vi "Update_Data_Packet_From_Processed_Bytes_Receiver.vi"(0 "Processed Bytes":u8[](array[numeric]), 1 "Receive count":u32, 2 "Receive interval (ms)":u32, 5 "Last Receive Time (ms)":u64, 11 "error in (no error)":errorcluster) -> (4 "Updated data packet":T1={"Packet"={"Raw Bytes"=[], "Checksum"=FALSE, "Direction"=enum."Transmit", "Processed Bytes"=[], "Node ID"=0, "Packet type"=enum."Connection Management", "Frame Data"=0, "Priority"=enum."LOW", "Frame ID"=0}, "Parameters"=[], "Last Received Time (ms)"=0, "Receive count"=0, "Transmit count"=0, "Transmit interval (ms)"=0, "Last Transmitted Time (ms)"=0, "Receive interval (ms)"=0, "Transmit_Mode"=enum."Disabled", "Transmit Enable"=FALSE, "Cyclic Transmit interval (ms)"=0}, 6 "Data Packets Out":T1[](array[typedef]), 15 "error out":errorcluster)   [LabVIEW 2017]
uses:
  Controls/Data Packets/Data_Packet.ctl
  Controls/Packet/Packet.ctl
  Controls/Packet/Packet_Direction.ctl
  Controls/Packet/Packet_Type.ctl
  Controls/Packet/Packet_Priority.ctl
  Controls/Data Packets/Parameter.ctl
  Controls/Data Packets/Parameter_Data_Type.ctl
  Controls/Data Packets/Data_Packet_Transmit_Mode.ctl
  Controls/Data Packets/Data_Packet_FGV_Commands.ctl
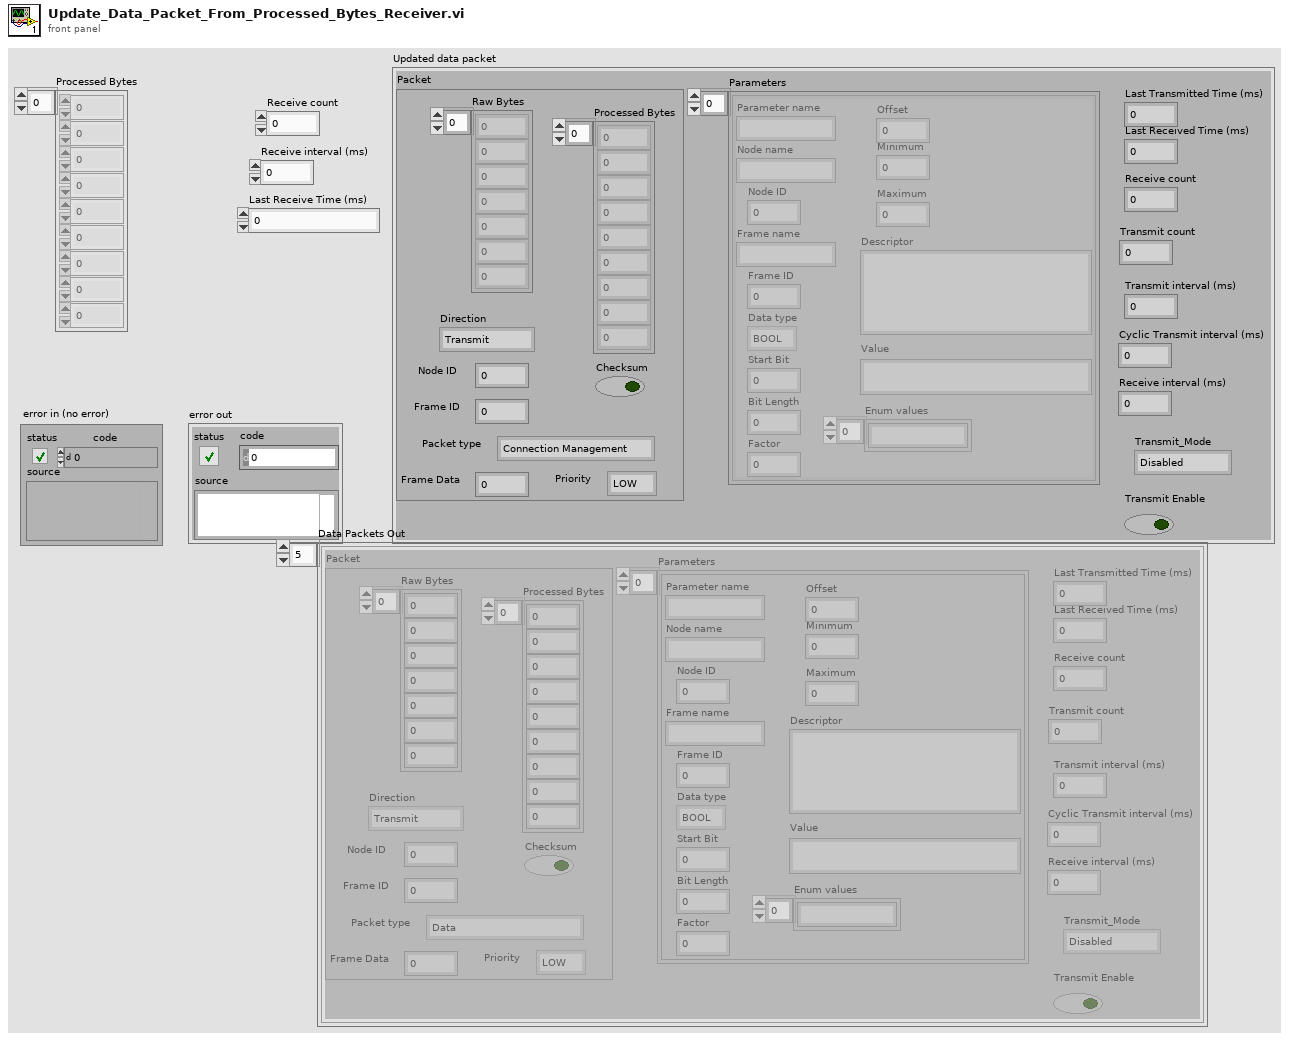
[diagram p1: front panel]
types:
  T1 = typedef "Data_Packet.ctl" = cluster{"Packet":T2, "Parameters":T6[], "Last Received Time (ms)":u64, "Receive count":i32, "Transmit count":i32, "Transmit interval (ms)":u32, "Last Transmitted Time (ms)":u64, "Receive interval (ms)":u32, "Transmit_Mode":T8, "Transmit Enable":bool, "Cyclic Transmit interval (ms)":u32}
  T2 = typedef "Packet.ctl" = cluster{"Raw Bytes":u8[], "Checksum":bool, "Direction":T3, "Processed Bytes":u8[], "Node ID":u8, "Packet type":T4, "Frame Data":u32, "Priority":T5, "Frame ID":u8}
  T3 = typedef "Packet_Direction.ctl" = enum16{"Transmit", "Receive", "Bidirectional"}
  T4 = typedef "Packet_Type.ctl" = enum16{"Data", "Connection Management", "Remote Request", "Error/Status"}
  T5 = typedef "Packet_Priority.ctl" = enum16{"LOW", "HIGH"}
  T6 = typedef "Parameter.ctl" = cluster{"Parameter name":string, "Node name":string, "Node ID":u8, "Frame name":string, "Frame ID":u8, "Data type":T7, "Start Bit":i32, "Bit Length":i32, "Factor":dbl, "Offset":dbl, "Minimum":dbl, "Maximum":dbl, "Descriptor":string, "Enum values":string[], "Value":string}
  T7 = typedef "Parameter_Data_Type.ctl" = enum16{"BOOL", "UNSIGNED", "SIGNED", "FLOAT32", "ENUM"}
  T8 = typedef "Data_Packet_Transmit_Mode.ctl" = enum16{"Disabled", "Single", "Cyclic"}
  T9 = typedef "Data_Packet_FGV_Commands.ctl" = enum16{"Update all parameters from data packets", "Update Packet", "Load", "Read Packet Parameters", "Write Packet Parameters", "Read Packet Parameter", "Write Packet Parameter", "Read Data Packets", "Read Data Packet", "Read Data Packet by Parameter Name", "Get Parameter Node and Frame ID", "Read Data Packet from Node ID and Frame ID"}
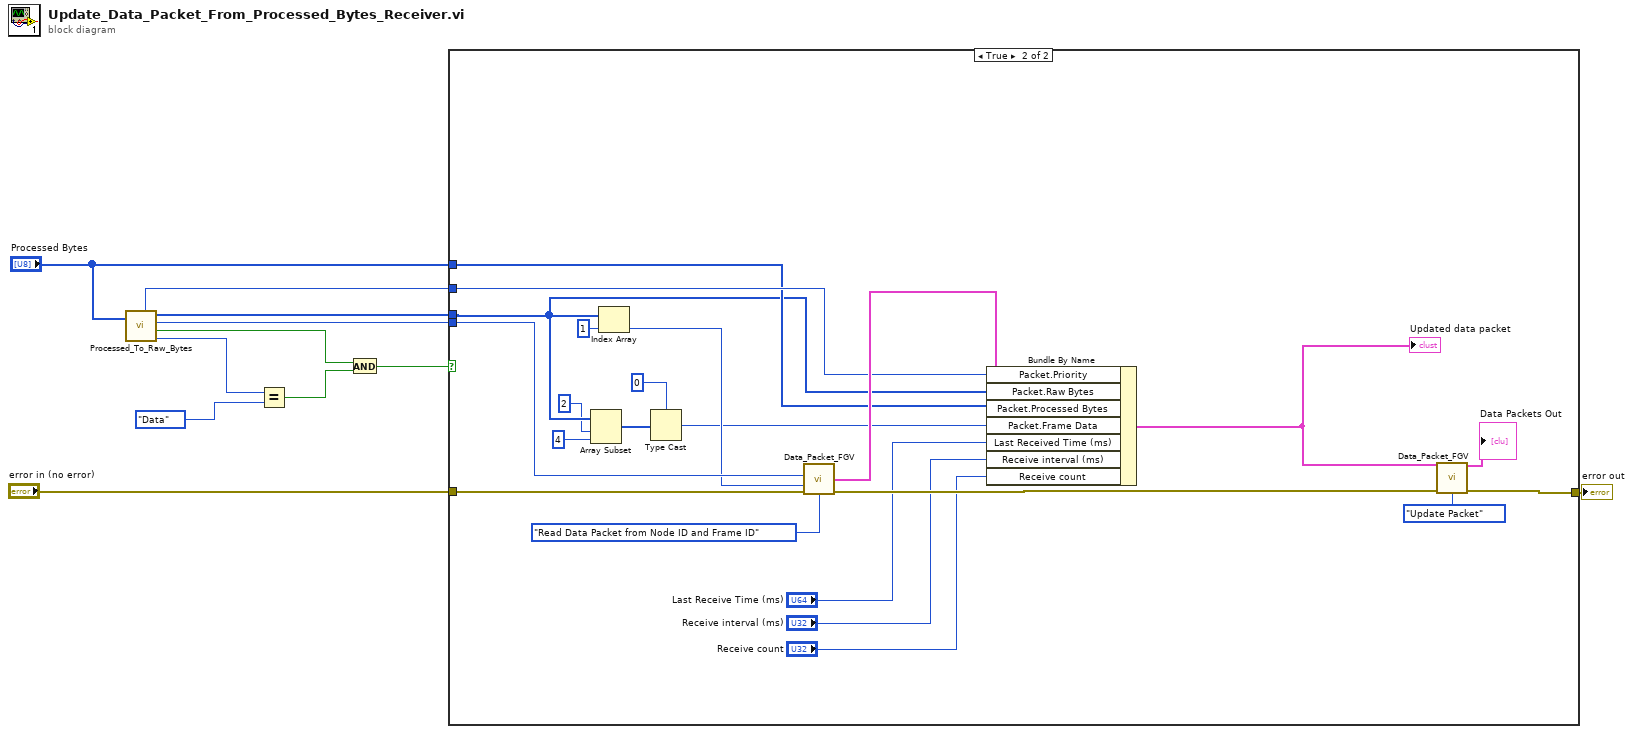
[diagram p0: block diagram]
diagram:
  n1 = call "Processed_To_Raw_Bytes.vi"("Processed Bytes"="Processed Bytes") -> ("Packet Type"=w10:T4, "Checksum"=w4:bool, "Node ID"=w8:u8, "Raw Bytes"=w7:u8[], "Priority"=w5:T5)  [unwired: 1 in]
  n2 = Equal?(x=w10, y=Packet_Type."Data") -> (x = y?=w3:bool)
  n3 = And(x=w4, y=w3) -> (x .and. y?=w2:bool)
  n4 = case shown="True" w2 {
    tunnel: "error in (no error)" -> [w12 w33]
    tunnel: w8 -> [_ w32]
    tunnel: w7 -> [_ w26]
    tunnel: "Processed Bytes" -> [_ w27]
    tunnel: w5 -> [_ w28]
    tunnel: [w12 w18] -> w1
    frame False {
    }
    frame True {
      n5 = Array Subset(array=w26, index=2, length=4) -> (w23:u8[])
      n6 = Index Array(array=w26, index=1) -> (element=w30:u8)
      n7 = Type Cast(type=u32 0, x=w23) -> (*(type *) &x=w21:u32)
      n8 = call "Data_Packet_FGV.vi"("Node ID"=w32, "Frame ID"=w30, "error in (no error)"=w33, "Commands"=Data_Packet_FGV_Commands."Read Data Packet from Node ID and Frame ID") -> ("Data_Packet out"=w29:T1, "error out"=w20:errorcluster)  [unwired: 6 in, 4 out]
      n9 = Bundle By Name(cluster=w29, "Packet.Priority"=w28, "Packet.Raw Bytes"=w26, "Packet.Processed Bytes"=w27, "Packet.Frame Data"=w21, "Last Received Time (ms)"="Last Receive Time (ms)", "Receive interval (ms)"="Receive interval (ms)", "Receive count"="Receive count") -> (w13:T1)
      "Updated data packet" <- w13
      n10 = call "Data_Packet_FGV.vi"("Data_Packet In"=w13, "error in (no error)"=w20, "Commands"=Data_Packet_FGV_Commands."Update Packet") -> ("Data Packets Out"=→"Data Packets Out":T1[], "error out"=w18:errorcluster)  [unwired: 7 in, 4 out]
    }
  }
  "error out" <- w1
